vi "Obtain Session.vi"(0 "Session  Name ()":string, 11 "error in (no error)":errorcluster) -> (4 "Session Handle":T1, 15 "error out":errorcluster)   [LabVIEW 2019, in "SmartScopeDriver.lvclass"]
doc: "This function initializes the measurement\n\nPass the function a name to obtain an active measurement handle"
uses:
  SmartScopeDriver.lvclass
  <userlib>/_Session Fwk/Session - Root.lvclass
  C:/Program Files (x86)/National Instruments/LabVIEW 2019/user.lib/_Session Fwk/Session - Root.lvclass
  Typedefs/Session Handle.ctl
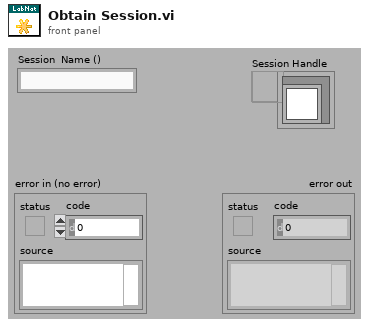
[diagram p1: front panel]
types:
  T1 = typedef "SmartScopeDriver.lvclass/Session Handle.ctl" = refnum<data-value>
  T2 = typedef "Session - Root.lvclass/Session Handle.ctl" = refnum<data-value>
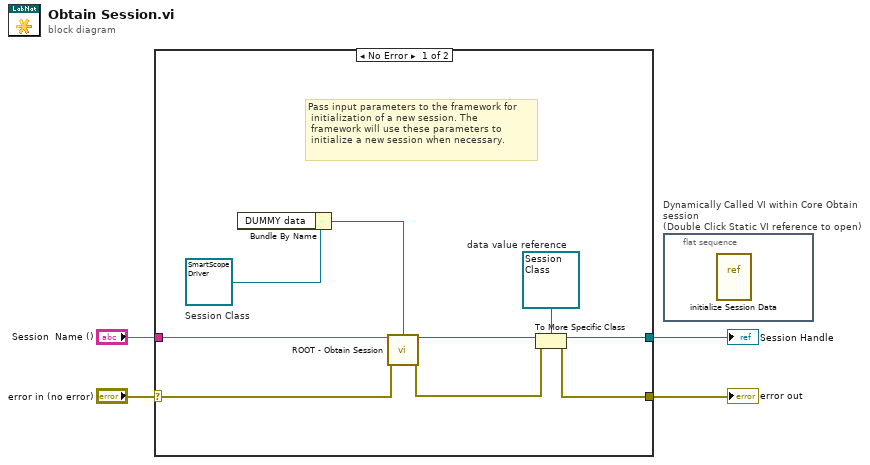
[diagram p0: block diagram]
diagram:
  n1 = case shown="No Error" "error in (no error)" {
    selector: "error in (no error)" -> [w12 w14]
    tunnel: [w9 w14] -> w3
    tunnel: [w11 _] -> w1
    tunnel: "Session  Name ()" -> [w13 _]
    frame No Error {
      w5 = refnum<data-value> refnum  # data value reference
      w6 = refnum<class "SmartScopeDriver.lvclass"> refnum  # Session Class
      # "Pass input parameters to the framework for\n initialization of a new session. The\n framework will use these parameters to\n initialize a new session when necessary."
      n2 = Bundle By Name(cluster=w6) -> (w7:refnum<class "SmartScopeDriver.lvclass">)  [unwired: 1 in]
      n3 = call <userlib>:"ROOT - Obtain Session.vi"("Session Name ()"=w13, "OBJ - Session"=w7, "error in (no error)"=w12) -> ("Session Handle"=w8:T2, "error out"=w10:errorcluster)  [unwired: 10 in, 1 out]
      n4 = To More Specific Class(target class=w5, reference=w8, error in=w10) -> (specific class reference=w11:refnum<data-value>, error out=w9:errorcluster)
    }
    frame Error {
    }
  }
  "error out" <- w3
  "Session Handle" <- w1
  n5 = flat-sequence "Dynamically Called VI within Core Obtain session\n(Double Click Static VI reference to open)" {
    frame #0 {
      n6 = vi-ref "initialize Session Data.vi"() -> ()  [unwired: 1 out]
    }
  }
